vi "MIDI Handler.vi"(8 "Error In":errorcluster, 11 "App-Data In":T2={"Console log"="", "GUI_Events"={"To_GUI-Producer"=refnum, "To_GUI-Error_message"=refnum, "To_GUI-msg_list"=refnum, "To_GUI-Session"=refnum, "To_GUI-Pre-Session"=refnum, "To_GUI-Consumer"=refnum}, "Function_Queue"={"Queue_MIDI_Handler"=refnum, "Queue_Session"=refnum, "Queue_Producer"=refnum, "Queue_Consumer"=refnum}, "Timout-Time[ms]"=0, "MIDI-Messages"=[], "Com Session State"=enum."Active Session", "Result Data"={"Diff"=[], "Tx Byte"=[], "Rx Byte"=[], "Send Log"=[], "Parsed Data"={"Tx MIDI Tag"=[], "Tx MIDI Parsed Data"=[], "Tx Error"=[], "Tx Running States"=[], "Rx MIDI Tag"=[], "Rx MIDI Parsed Data"=[], "Rx Error"=[], "Rx Running States"=[], "Diff"=[]}}, "Get #"=[], "CPU(ms)"=0}) -> (0 "Error Out":errorcluster, 3 "MIDI Data Out":T11)   [LabVIEW 2019]
doc: "Loads inn textfiles containing MIDI-events and messages, concatenates and generates a message string to send."
uses:
  Common/Controls/Application_Data.ctl
  Common/Controls/App_Events.ctl
  Common/Controls/App_Queues.ctl
  Common/Controls/Application_Message.ctl
  Common/Controls/Application_State.ctl
  Controls/MIDI-Message_Array.ctl
  Controls/MIDI-Message_Cluster.ctl
  Controls/Meta_Commands.ctl
  Producer/Controls/Session_State.ctl
  Consumer/Controls/Consumer_Result.ctl
  Consumer/Controls/Parsed_Data.ctl
  Controls/MIDI-Data.ctl
  <vilib>/Utility/error.llb/DialogType.ctl
panel:
  in  "Control Tab":T1(tab)
  in  "Available Messages":i32(listbox)
  out "Log":string
  out "Error Message":string
  in  "Tabs Visible":bool=TRUE
  out "VI-filename":string
  out "VI Path":path
  out "Code Size":u32
  out "Revision Number":u32
  in  "Tool Bar:Visible":bool
  out "VI-Name":string
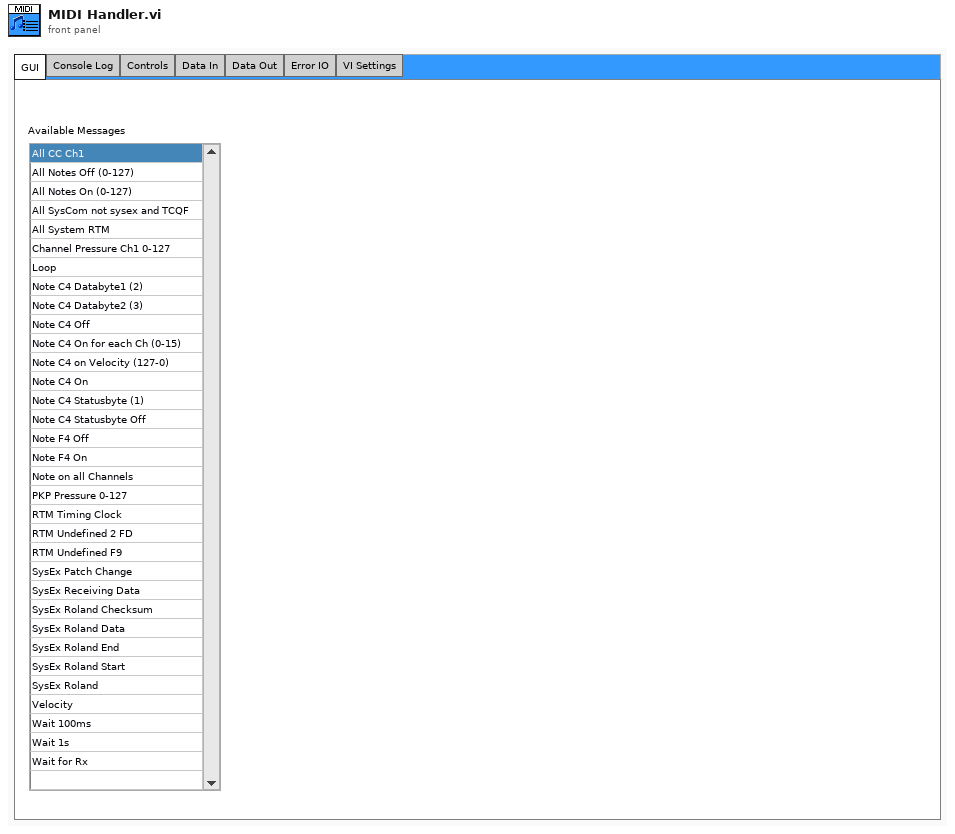
[diagram p1: front panel]
types:
  T1 = enum32{"GUI", "Console Log", "Controls", "Data In", "Data Out", "Error IO", "VI Settings"}
  T2 = typedef "Application_Data.ctl" = cluster{"Console log":string, "GUI_Events":T3, "Function_Queue":T4, "Timout-Time[ms]":i32, "MIDI-Messages":T5, "Com Session State":T8, "Result Data":T9, "Get #":bool[], "CPU(ms)":u32}
  T3 = typedef "App_Events.ctl" = cluster{"To_GUI-Producer":refnum<user-event>, "To_GUI-Error_message":refnum<user-event>, "To_GUI-msg_list":refnum<user-event>, "To_GUI-Session":refnum<user-event>, "To_GUI-Pre-Session":refnum<user-event>, "To_GUI-Consumer":refnum<user-event>}
  T4 = typedef "App_Queues.ctl" = cluster{"Queue_MIDI_Handler":refnum<queue>, "Queue_Session":refnum<queue>, "Queue_Producer":refnum<queue>, "Queue_Consumer":refnum<queue>}
  T5 = typedef "MIDI-Message_Array.ctl" = T6[]
  T6 = typedef "MIDI-Message_Cluster.ctl" = cluster{"Message Name":string, "Meta value":i32, "Datastring":string, "Datatype":T7}
  T7 = typedef "Meta_Commands.ctl" = enum16{"No Data", "Pause", "Loop", "Wait for Rx", "Delay", "Break", "MIDI"}
  T8 = typedef "Session_State.ctl" = enum16{"Wait to begin", "Active Session", "Pause", "Wait for Response", "Stop", "Restart", "Inspect", "Exit"}
  T9 = typedef "Consumer_Result.ctl" = cluster{"Diff":bool[], "Tx Byte":string[], "Rx Byte":string[], "Send Log":string[], "Parsed Data":T10}
  T10 = typedef "Parsed_Data.ctl" = cluster{"Tx MIDI Tag":string[], "Tx MIDI Parsed Data":string[], "Tx Error":bool[], "Tx Running States":string[], "Rx MIDI Tag":string[], "Rx MIDI Parsed Data":string[], "Rx Error":bool[], "Rx Running States":string[], "Diff":bool[]}
  T11 = typedef "MIDI-Data.ctl" = cluster{"Console log":string, "Payload":variant, "MIDI Message Array":T5, "Timout-Time[ms]":i32, "Queue_MIDI_Handler":refnum<queue>, "To_GUI-Error_message":refnum<user-event>, "To_GUI-msg_list":refnum<user-event>, "CPU(ms)":u32}
  T12 = typedef "DialogType.ctl" = u16
  T13 = typedef "Application_State.ctl" = enum16{"Idle", "Initiate", "MH Load Messages", "Prepare for Tx", "Settings", "Com Session", "Receive", "Data", "Uninitialize", "Quit Message", "Export Send"}
  T14 = typedef "Application_Message.ctl" = cluster{"Application State":T13, "Payload":variant}
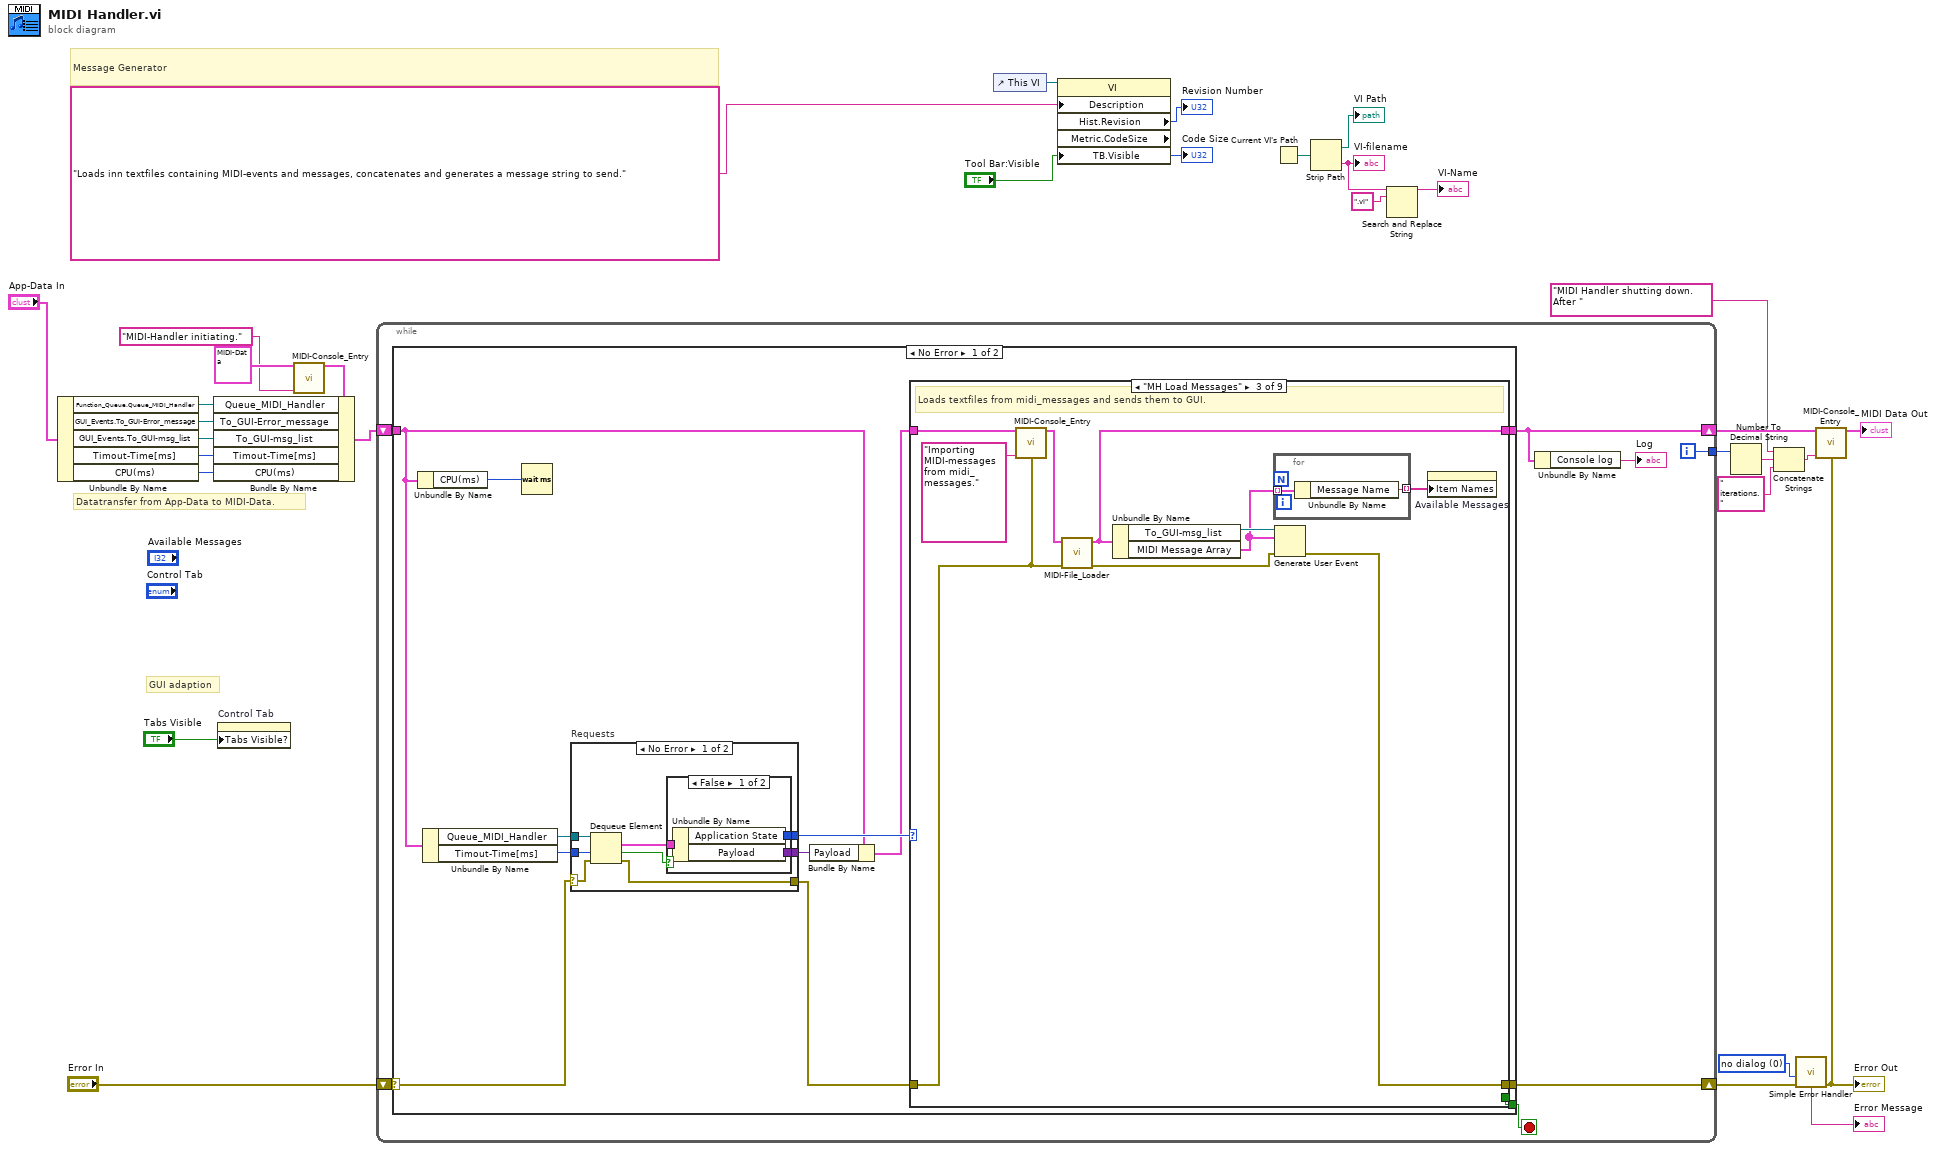
[diagram p0: block diagram]
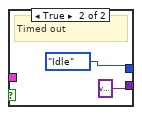
[diagram p2: hidden frame]
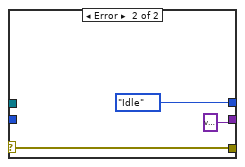
[diagram p3: hidden frame]
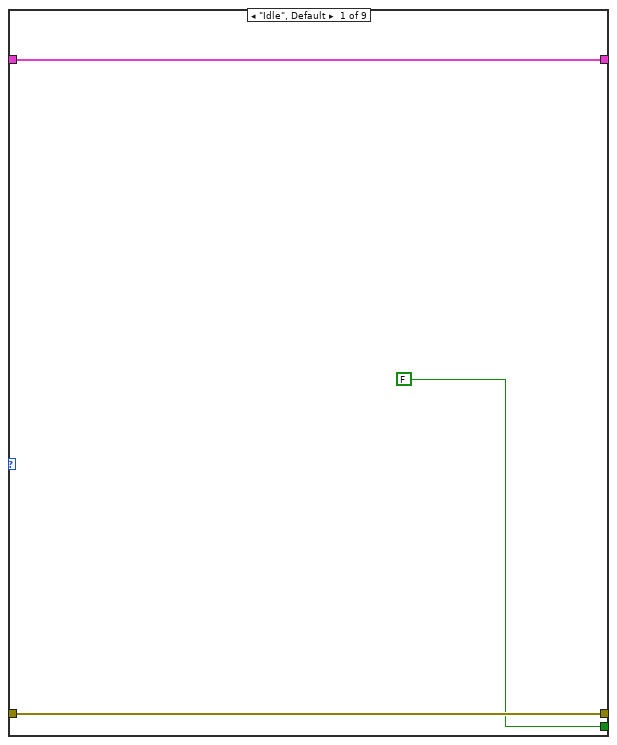
[diagram p4: hidden frame]
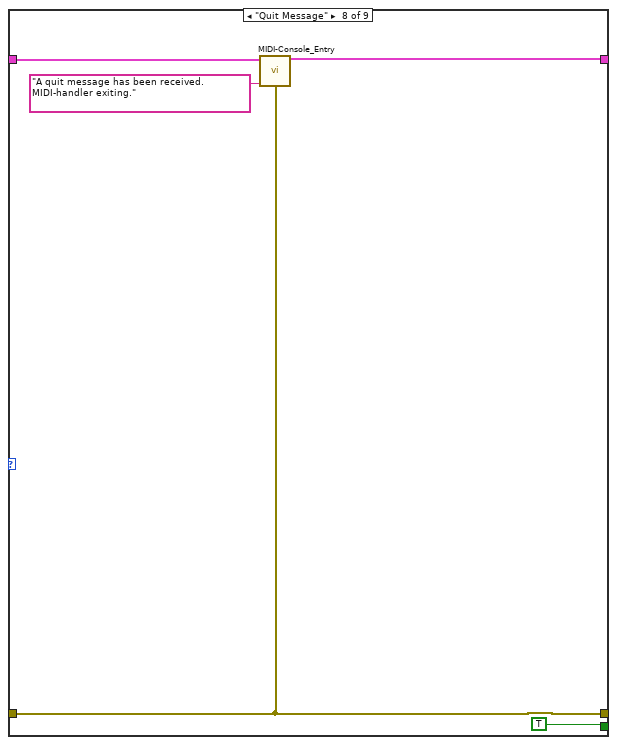
[diagram p10: hidden frame]
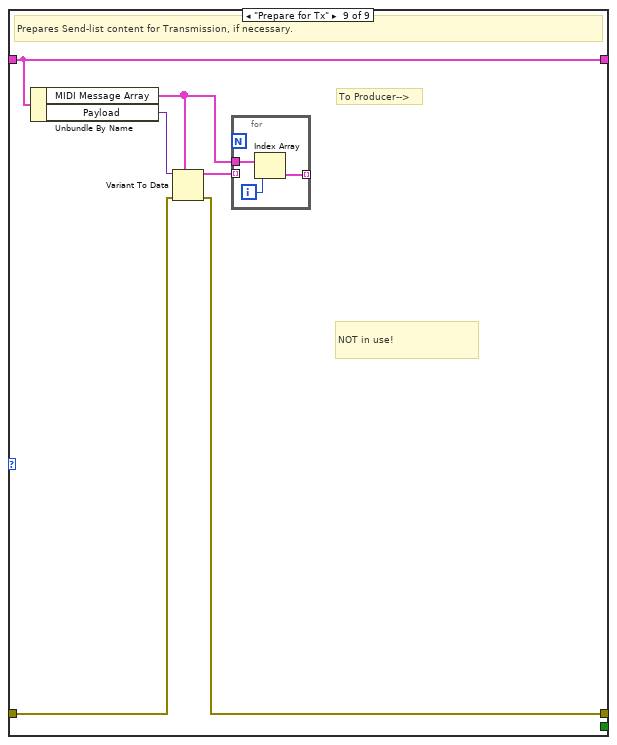
[diagram p11: hidden frame]
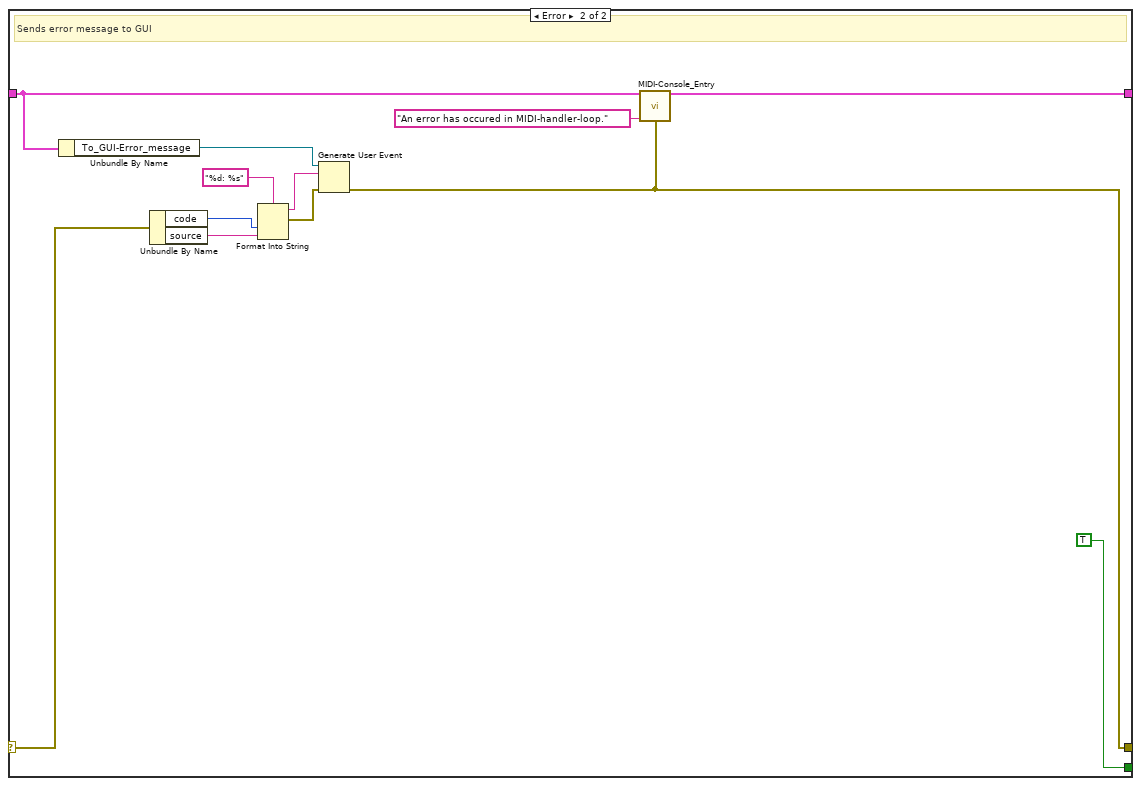
[diagram p12: hidden frame]
diagram:
  w22 = T12 0 items=["no dialog", "OK message", "continue or stop message", "OK message + warnings", "continue/stop + warnings"] ("type of dialog (OK msg:1)")
  # "GUI adaption"
  # "Datatransfer from App-Data to MIDI-Data."
  # "Message Generator"
  n1 = Unbundle By Name("App-Data In") -> ("Function_Queue.Queue_MIDI_Handler"=w18:refnum<queue>, "GUI_Events.To_GUI-Error_message"=w20:refnum<user-event>, "GUI_Events.To_GUI-msg_list"=w15:refnum<user-event>, "Timout-Time[ms]"=w16:i32, "CPU(ms)"=w12:u32)
  n2 = property on="Control Tab" class="TabCtl (strict)"("Tabs Visible?"="Tabs Visible") -> ()  [unwired: 2 in, 2 out]
  n3 = call "MIDI-Console_Entry.vi"("Data In"=T11 {"Console log"="", "Payload"=variant, "MIDI Message Array"=[], "Timout-Time[ms]"=0, "Queue_MIDI_Handler"=refnum, "To_GUI-Error_message"=refnum, "To_GUI-msg_list"=refnum, "CPU(ms)"=0}, "Console Entry"="MIDI-Handler initiating.") -> ("Data Out"=w3:T11)  [unwired: 13 in]
  n4 = Bundle By Name(cluster=w3, "Queue_MIDI_Handler"=w18, "To_GUI-Error_message"=w20, "To_GUI-msg_list"=w15, "Timout-Time[ms]"=w16, "CPU(ms)"=w12) -> (w13:T11)
  n5 = while {
    shift-right: [w36] -> w10
    shift-left: w13 -> [w40]
    shift-right: [w38] -> w14
    shift-left: "Error In" -> [w39]
    tunnel: [w34] -> w5
    i -> [w34]
    stop <- w37 stop-if-true
    n6 = case shown="No Error" w39 {
      selector: w39 -> [w48 w117]
      tunnel: w40 -> [w42 w111]
      tunnel: [w44 w110] -> w36
      tunnel: [w52 w109] -> w38
      tunnel: [w43 TRUE] -> w37
      frame No Error {
        n7 = Unbundle By Name(w42) -> ("CPU(ms)"=w41:u32)
        n8 = Unbundle By Name(w42) -> ("Queue_MIDI_Handler"=w51:refnum<queue>, "Timout-Time[ms]"=w50:i32)
        n9 = Wait (ms)(milliseconds to wait=w41) -> ()  [unwired: 1 out]
        n10 = case "Requests" shown="No Error" w48 {
          selector: w48 -> [w58 w67]
          tunnel: w51 -> [w60 _]
          tunnel: w50 -> [w59 _]
          tunnel: [w53 w67] -> w49
          tunnel: [w55 Application_State."Idle" ("Message_Types")] -> w47
          tunnel: [w54 variant ("Payload")] -> w46
          frame No Error {
            n11 = Dequeue Element(queue=w60, timeout in ms (-1)=w59, error in (no error)=w58) -> (element=w56:T14, timed out?=w57:bool, error out=w53:errorcluster)  [unwired: 1 out]
            n12 = case shown="False" w57 {
              tunnel: w56 -> [w63 _]
              tunnel: [w62 Application_State."Idle" ("Message_Types")] -> w55
              tunnel: [w61 variant ("Payload")] -> w54
              frame False {
                n13 = Unbundle By Name(w63) -> ("Application State"=w62:T13, "Payload"=w61:variant)
              }
              frame True {
                # "Timed out"
              }
            }
          }
          frame Error {
          }
        }
        n14 = Bundle By Name(cluster=w42, "Payload"=w46) -> (w45:T11)
        n15 = case shown="\"MH Load Messages\"" w47 {
          tunnel: w49 -> [w70 w72 w75 w86 w88 w90 w92 w94 w103]
          tunnel: w45 -> [w71 w73 w76 w87 w89 w91 w93 w97 w100]
          tunnel: [w70 w72 w78 w86 w88 w90 w92 w94 w99] -> w52
          tunnel: [w71 w73 w82 w87 w89 w91 w93 w96 w100] -> w44
          tunnel: [FALSE _ _ _ _ _ _ TRUE _] -> w43
          frame "Idle", Default {
          }
          frame "Initiate" {
          }
          frame "MH Load Messages" {
            # "Loads textfiles from midi_messages and sends them to GUI."
            n16 = call "MIDI-Console_Entry.vi"("Data In"=w76, "Console Entry"="Importing MIDI-messages from midi_messages.", "Error In"=w75) -> ("Data Out"=w77:T11)  [unwired: 12 in]
            n17 = call "MIDI-File_Loader.vi"("Error In"=w75, "MIDI-Data In"=w77) -> ("Error Out"=w79:errorcluster, "MIDI-Data Out"=w82:T11)  [unwired: 8 in]
            n18 = Unbundle By Name(w82) -> ("To_GUI-msg_list"=w83:refnum<user-event>, "MIDI Message Array"=w81:T5)
            n19 = for {
              tunnel: w81 -> [w85] mode=indexing
              tunnel: [w84] -> w80 mode=indexing
              n20 = Unbundle By Name(w85) -> ("Message Name"=w84:string)
            }
            n21 = Generate User Event(user event=w83, event data cluster=w81, error in=w79) -> (error out=w78:errorcluster)  [unwired: 1 in, 1 out]
            n22 = property on="Available Messages" class="LstBox (strict)"("Item Names"=w80) -> ()  [unwired: 2 in, 2 out]
          }
          frame "Settings" {
          }
          frame "Com Session" {
          }
          frame "Receive" {
          }
          frame "Data" {
          }
          frame "Quit Message" {
            n23 = call "MIDI-Console_Entry.vi"("Data In"=w97, "Console Entry"="A quit message has been received. MIDI-handler exiting.", "Error In"=w94) -> ("Data Out"=w96:T11)  [unwired: 12 in]
          }
          frame "Prepare for Tx" {
            # "NOT in use!"
            # "To Producer-->"
            # "Prepares Send-list content for Transmission, if necessary."
            n24 = Unbundle By Name(w100) -> ("MIDI Message Array"=w101:T5, "Payload"=w104:variant)
            n25 = Variant To Data(error in=w103, type=w101, Variant=w104) -> (data=w102:T5, error out=w99:errorcluster)
            n26 = for {
              tunnel: w102 -> [_] mode=indexing
              tunnel: w101 -> [w107]
              tunnel: [w106] -> _ mode=indexing
              i -> [w105]
              n27 = Index Array(array=w107, index=w105) -> (element=w106:T6)
            }
          }
        }
      }
      frame Error {
        # "Sends error message to GUI"
        n28 = Unbundle By Name(w111) -> ("To_GUI-Error_message"=w118:refnum<user-event>)
        n29 = Unbundle By Name(w117) -> ("code"=w116:i32, "source"=w115:string)
        n30 = Format Into String(format string="%d: %s", w116, w115) -> (resulting string=w113:string, error out=w112:errorcluster)  [unwired: 2 in]
        n31 = Generate User Event(user event=w118, event data cluster=w113, error in=w112) -> (error out=w109:errorcluster)  [unwired: 1 in, 1 out]
        n32 = call "MIDI-Console_Entry.vi"("Data In"=w111, "Console Entry"="An error has occured in MIDI-handler-loop.", "Error In"=w109) -> ("Data Out"=w110:T11)  [unwired: 12 in]
      }
    }
    n33 = Unbundle By Name(w36) -> ("Console log"=→"Log":string)
  }
  n34 = control-ref of="This VI"() -> (w28:refnum<vi>)
  n35 = property class="VI"(reference=w28, "Description"="Loads inn textfiles containing MIDI-events and messages, concatenates and generates a message string to send.", "TB.Visible"="Tool Bar:Visible") -> ("Hist.Revision"=→"Revision Number":u32, "Metric.CodeSize"=→"Code Size":u32)  [unwired: 1 in, 2 out]
  n36 = Current VI's Path() -> (path=w33:path)
  n37 = Strip Path(path=w33) -> (stripped path=→"VI Path":path, name=w25:string)
  "VI-filename" <- w25
  n38 = Search and Replace String(input string=w25, search string=".vi") -> (result string=→"VI-Name":string)  [unwired: 6 in, 3 out]
  n39 = Number To Decimal String(number=w5) -> (decimal integer string=w6:string)  [unwired: 1 in]
  n40 = Concatenate Strings("MIDI Handler shutting down. After " ("Console Entry"), w6, " iterations." ("string")) -> (w8:string)
  n41 = call <vilib>:"Simple Error Handler.vi"("type of dialog (OK msg:1)"=w22, "error in (no error)"=w14) -> ("error out"=w9:errorcluster, "message"=→"Error Message":string)  [unwired: 3 in, 3 out]
  "Error Out" <- w9
  n42 = call "MIDI-Console_Entry.vi"("Data In"=w10, "Console Entry"=w8, "Error In"=w9) -> ("Data Out"=→"MIDI Data Out":T11)  [unwired: 12 in]
